vi "(SubVI)Scope_Trigger Counting.vi"(7 "Init":bool, 9 "Sampling Time":dbl format="%#_13g", 10 "Trigger Setting":T1 {"Capture Delay (sec.)" min=0.0 max=5.0; "Pre-Trigger (sec.)" max=10.0}, 11 "Scope Data In":i16[][](array[numeric])) -> (1 "Stop":bool, 2 "Trigger Count":u32, 3 "Scope Data Out":i16[][](array[numeric]))   [LabVIEW 2020]
uses:
  Log/Controls/(Ctrl)Scope_Log_Trigger_Setting.ctl
  Log/Controls/(Ctrl)Scope_Log_Trigger_Type.ctl
  Log/Controls/(Ctrl)Scope_Log_Trigger_Edge.ctl
  Log/Controls/(Ctrl)Scope_Log_Trigger_Edge_Slope.ctl
  Log/Controls/(Ctrl)Scope_Log_Trigger_Window.ctl
  Log/Controls/(Ctrl)Scope_Log_Trigger_Window_When.ctl
  Log/Controls/(Ctrl)Scope_Log_Trigger_Mode.ctl
  a86a7f54-a3bc-428c-973f-614ca024c295.vi
  0bc404e9-e659-4e8a-81b1-d0e0b6e0689e.vi
  <vilib>/Comparison/Equal/Equal Functor/Equal Functor.lvclass
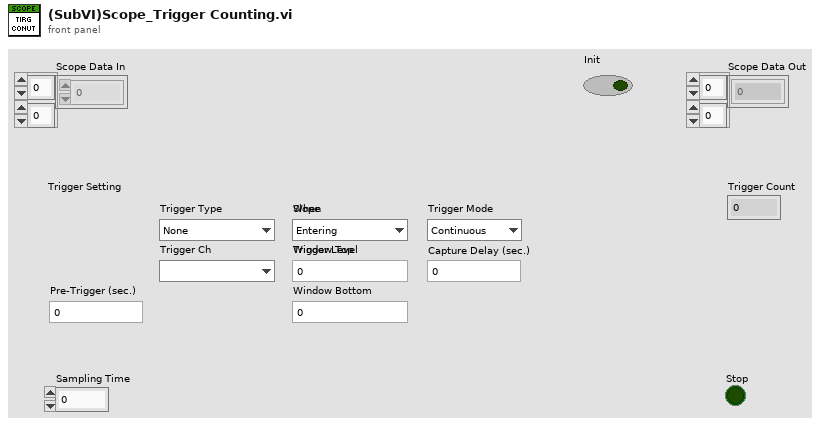
[diagram p1: front panel]
types:
  T1 = typedef "(Ctrl)Scope_Log_Trigger_Setting.ctl" = cluster{"Trigger Type":T2, "Trigger Ch":u16, "Pre-Trigger (sec.)":dbl, "Trigger_Edge":T3, "Trigger_Window":T5, "Trigger Mode":T7, "Capture Delay (sec.)":dbl}
  T2 = typedef "(Ctrl)Scope_Log_Trigger_Type.ctl" = enum16{"None", "Edge", "Window"}
  T3 = typedef "(Ctrl)Scope_Log_Trigger_Edge.ctl" = cluster{"Slope":T4, "Trigger Level":i16}
  T4 = typedef "(Ctrl)Scope_Log_Trigger_Edge_Slope.ctl" = enum16{"Rising", "Falling"}
  T5 = typedef "(Ctrl)Scope_Log_Trigger_Window.ctl" = cluster{"When":T6, "Window Top":i16, "Window Bottom":i16}
  T6 = typedef "(Ctrl)Scope_Log_Trigger_Window_When.ctl" = enum16{"Entering", "Leaving"}
  T7 = typedef "(Ctrl)Scope_Log_Trigger_Mode.ctl" = enum16{"Continuous", "Capture"}
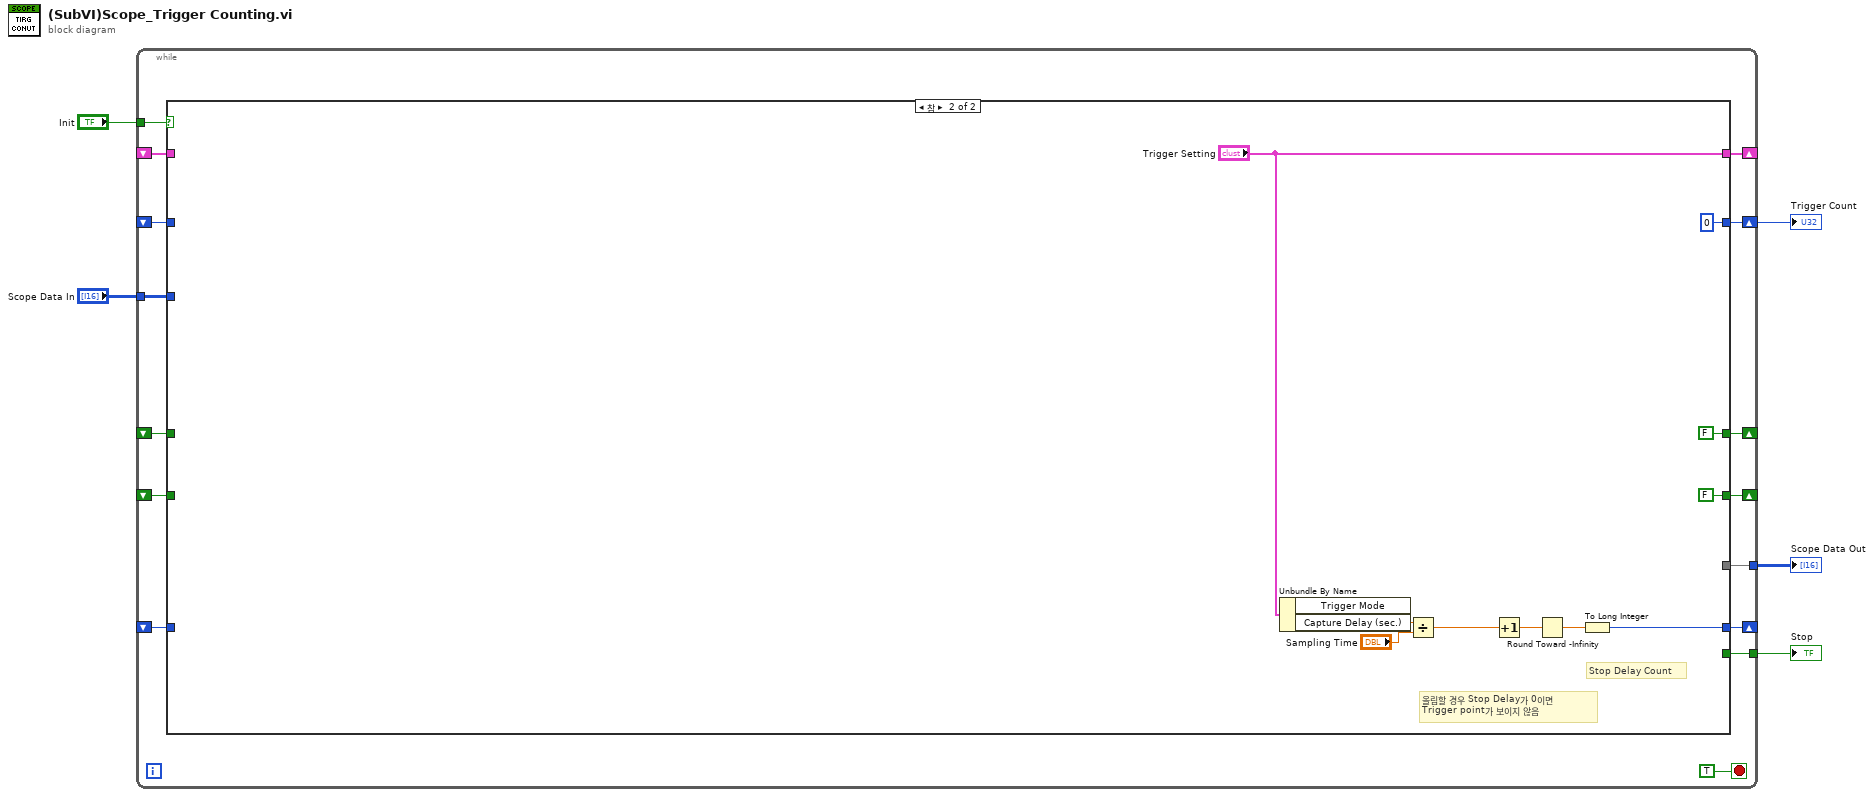
[diagram p0: block diagram]
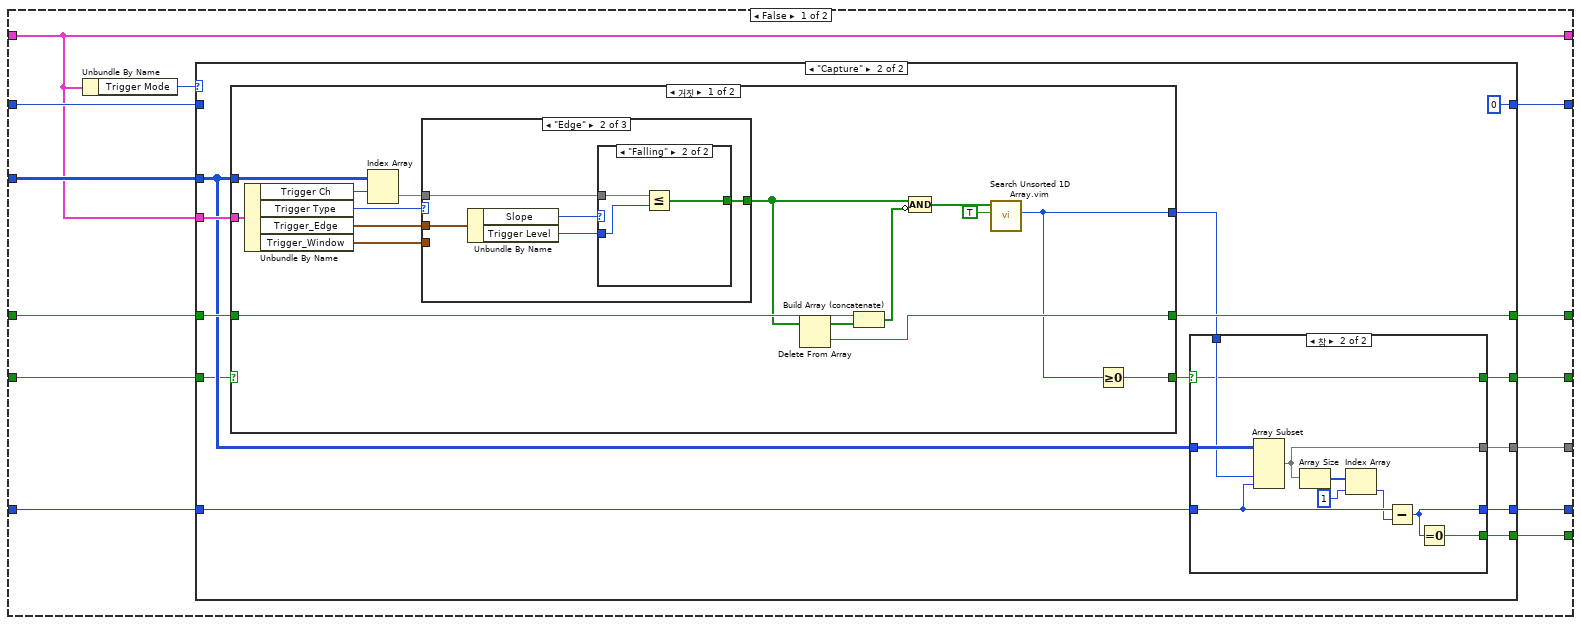
[diagram p2: hidden frame]
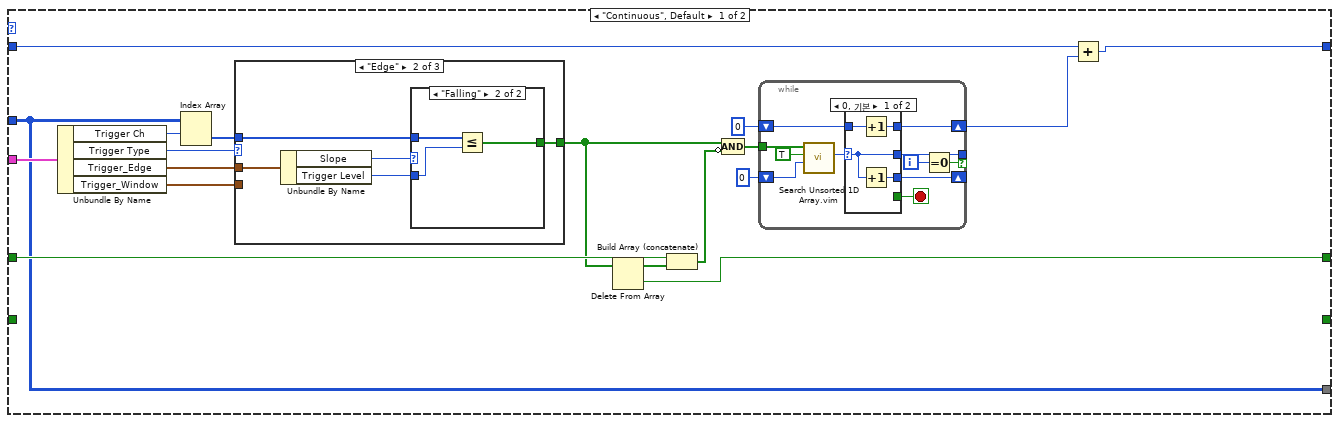
[diagram p3: hidden frame]
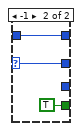
[diagram p4: hidden frame]
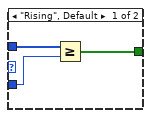
[diagram p6: hidden frame]
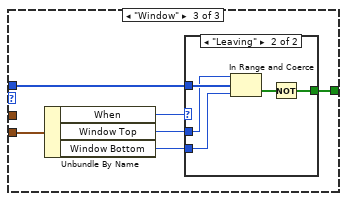
[diagram p7: hidden frame]
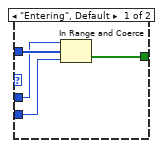
[diagram p8: hidden frame]
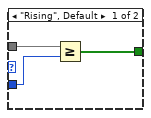
[diagram p10: hidden frame]
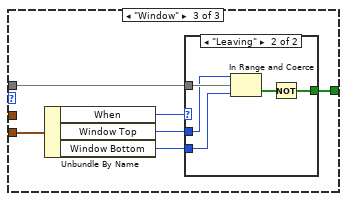
[diagram p11: hidden frame]
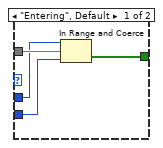
[diagram p12: hidden frame]
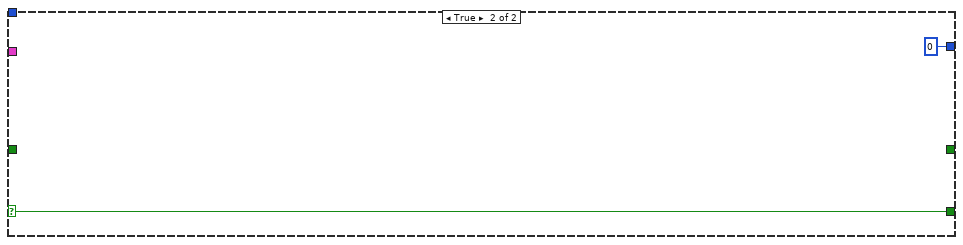
[diagram p13: hidden frame]
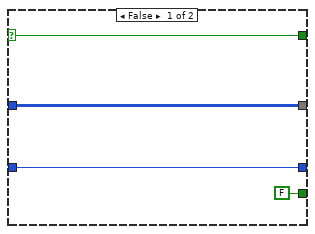
[diagram p14: hidden frame]
diagram:
  n1 = while {
    shift-right: [w20] -> _
    shift-left: _ -> [w19]
    tunnel: "Scope Data In" -> [w15]
    tunnel: "Init" -> [w14]
    shift-right: [w17] -> w1
    shift-left: _ -> [w13]
    shift-right: [w12] -> _
    shift-left: _ -> [w11]
    shift-right: [w10] -> _
    shift-left: _ -> [w16]
    shift-right: [w9] -> _
    shift-left: _ -> [w8]
    tunnel: [w7] -> w3
    tunnel: [w6] -> w2
    stop <- TRUE stop-if-true
    n2 = case shown="참" w14 {
      tunnel: [w33 FALSE ("Window Top")] -> w20
      tunnel: w19 -> [w32 _]
      tunnel: [w30 u32 0] -> w17
      tunnel: w16 -> [w22 _]
      tunnel: w15 -> [w27 _]
      tunnel: w13 -> [w31 _]
      tunnel: [w29 FALSE] -> w12
      tunnel: w11 -> [w28 _]
      tunnel: [w22 "Trigger Setting"] -> w10
      tunnel: [w24 w170] -> w9
      tunnel: w8 -> [w26 _]
      tunnel: [w25 _] -> w7
      tunnel: [w23 _] -> w6
      frame False {
        n3 = Unbundle By Name(w22) -> ("Trigger Mode"=w21:T7)
        n4 = case shown="\"Capture\"" w21 {
          tunnel: [w44 w108] -> w33
          tunnel: w32 -> [w43 w107]
          tunnel: w31 -> [w39 _]
          tunnel: [w38 u32 0] -> w30
          tunnel: [_ w106] -> w29
          tunnel: w28 -> [_ w97]
          tunnel: w22 -> [w36 w104]
          tunnel: w27 -> [w34 w103]
          tunnel: w26 -> [_ w102]
          tunnel: [w34 w101] -> w25
          tunnel: [_ w100] -> w24
          tunnel: [_ w99] -> w23
          frame "Continuous", Default {
            n5 = Unbundle By Name(w36) -> ("Trigger Ch"=w51:u16, "Trigger Type"=w50:T2, "Trigger_Edge"=w48:T3, "Trigger_Window"=w47:T5)
            n6 = Index Array(array=w34, index (row)=w51) -> (element=w49:i16[])  [unwired: 1 in]
            n7 = case shown="\"Edge\"" w50 {
              tunnel: w49 -> [_ w71 w84]
              tunnel: w48 -> [_ w74 _]
              tunnel: w47 -> [_ _ w82]
              tunnel: [_ w70 w83] -> w42
              frame "None" {
              }
              frame "Edge" {
                n8 = Unbundle By Name(w74) -> ("Slope"=w73:T4, "Trigger Level"=w72:i16)
                n9 = case shown="\"Falling\"" w73 {
                  tunnel: w72 -> [w76 w79]
                  tunnel: w71 -> [w77 w80]
                  tunnel: [w75 w78] -> w70
                  frame "Rising", Default {
                    n10 = Greater Or Equal?(x=w77, y=w76) -> (x >= y?=w75:bool[])
                  }
                  frame "Falling" {
                    n11 = Less Or Equal?(x=w80, y=w79) -> (x <= y?=w78:bool[])
                  }
                }
              }
              frame "Window" {
                n12 = Unbundle By Name(w82) -> ("When"=w86:T6, "Window Top"=w85:i16, "Window Bottom"=w81:i16)
                n13 = case shown="\"Leaving\"" w86 {
                  tunnel: w85 -> [w88 w93]
                  tunnel: w84 -> [w89 w94]
                  tunnel: [w90 w91] -> w83
                  tunnel: w81 -> [w87 w92]
                  frame "Entering", Default {
                    n14 = In Range and Coerce(upper limit=w88, x=w89, lower limit=w87) -> (In Range?=w90:bool[])  [unwired: 1 out]
                  }
                  frame "Leaving" {
                    n15 = In Range and Coerce(upper limit=w93, x=w94, lower limit=w92) -> (In Range?=w95:bool[])  [unwired: 1 out]
                    n16 = Not(x=w95) -> (.not. x?=w91:bool[])
                  }
                }
              }
            }
            n17 = Delete From Array(array=w42) -> (deleted portion=w44:bool, array with subset deleted=w45:bool[])  [unwired: 2 in]
            n18 = Build Array (concatenate)(w43, w45) -> (w46:bool[])
            n19 = Compound Arithmetic op=AND(w42, invert w46) -> (w41:bool[])
            n20 = while {
              tunnel: w41 -> [w61]
              shift-right: [w59] -> _
              shift-left: 0 -> [w58]
              shift-right: [w55] -> w37
              shift-left: u32 0 -> [w56]
              tunnel: [w54] -> _ if=w53
              i -> [w52]
              stop <- w57 stop-if-true
              n21 = call "Search Unsorted 1D Array.vim"("start index (0)"=w58, "element"=TRUE, "unsorted 1D array"=w61) -> ("index of element"=w60:i32)  [unwired: 8 in]
              n22 = case shown="0, 기본" w60 {
                selector: w60 -> [w63 w67]
                tunnel: [w66 _] -> w59
                tunnel: [_ TRUE] -> w57
                tunnel: w56 -> [w65 w68]
                tunnel: [w64 w68] -> w55
                tunnel: [w63 w67] -> w54
                frame 0, Default {
                  n23 = Increment(x=w65) -> (x+1=w64:u32)
                  n24 = Increment(x=w63) -> (x+1=w66:i32)
                }
                frame -1 {
                }
              }
              n25 = Equal To 0?(x=w52) -> (x = 0?=w53:bool)
            }
            n26 = Add(x=w39, y=w37) -> (x+y=w38:u32)
          }
          frame "Capture" {
            n27 = case shown="거짓" w97 {
              selector: w97 -> [_ w151]
              tunnel: [w117 _] -> w108
              tunnel: w107 -> [w116 _]
              tunnel: [w110 0 ("index of element")] -> w105
              tunnel: w104 -> [w113 _]
              tunnel: w103 -> [w112 _]
              tunnel: [w109 w151] -> w96
              frame False {
                n28 = Unbundle By Name(w113) -> ("Trigger Ch"=w124:u16, "Trigger Type"=w123:T2, "Trigger_Edge"=w121:T3, "Trigger_Window"=w120:T5)
                n29 = Index Array(array=w112, index (row)=w124) -> (element=w122:i16[])  [unwired: 1 in]
                n30 = case shown="\"Edge\"" w123 {
                  tunnel: w122 -> [_ w126 w139]
                  tunnel: w121 -> [_ w129 _]
                  tunnel: w120 -> [_ _ w137]
                  tunnel: [_ w125 w138] -> w115
                  frame "None" {
                  }
                  frame "Edge" {
                    n31 = Unbundle By Name(w129) -> ("Slope"=w128:T4, "Trigger Level"=w127:i16)
                    n32 = case shown="\"Falling\"" w128 {
                      tunnel: w127 -> [w131 w134]
                      tunnel: w126 -> [w132 w135]
                      tunnel: [w130 w133] -> w125
                      frame "Rising", Default {
                        n33 = Greater Or Equal?(x=w132, y=w131) -> (x >= y?=w130:bool[])
                      }
                      frame "Falling" {
                        n34 = Less Or Equal?(x=w135, y=w134) -> (x <= y?=w133:bool[])
                      }
                    }
                  }
                  frame "Window" {
                    n35 = Unbundle By Name(w137) -> ("When"=w141:T6, "Window Top"=w140:i16, "Window Bottom"=w136:i16)
                    n36 = case shown="\"Leaving\"" w141 {
                      tunnel: w140 -> [w143 w148]
                      tunnel: w139 -> [w144 w149]
                      tunnel: [w145 w146] -> w138
                      tunnel: w136 -> [w142 w147]
                      frame "Entering", Default {
                        n37 = In Range and Coerce(upper limit=w143, x=w144, lower limit=w142) -> (In Range?=w145:bool[])  [unwired: 1 out]
                      }
                      frame "Leaving" {
                        n38 = In Range and Coerce(upper limit=w148, x=w149, lower limit=w147) -> (In Range?=w150:bool[])  [unwired: 1 out]
                        n39 = Not(x=w150) -> (.not. x?=w146:bool[])
                      }
                    }
                  }
                }
                n40 = Delete From Array(array=w115) -> (deleted portion=w117:bool, array with subset deleted=w118:bool[])  [unwired: 2 in]
                n41 = Build Array (concatenate)(w116, w118) -> (w119:bool[])
                n42 = Compound Arithmetic op=AND(w115, invert w119) -> (w114:bool[])
                n43 = call "Search Unsorted 1D Array.vim"("element"=TRUE, "unsorted 1D array"=w114) -> ("index of element"=w110:i32)  [unwired: 9 in]
                n44 = Greater Or Equal To 0?(x=w110) -> (x >= 0?=w109:bool)
              }
              frame True {
              }
            }
            n45 = case shown="참" w96 {
              selector: w96 -> [w154 w160]
              tunnel: [w154 w160] -> w106
              tunnel: w105 -> [_ w164]
              tunnel: w103 -> [w155 w166]
              tunnel: w102 -> [w156 w165]
              tunnel: [w156 w158] -> w100
              tunnel: [w155 w163] -> w101
              tunnel: [FALSE w157] -> w99
              frame False {
              }
              frame True {
                n46 = Array Subset(array=w166, index (col)=w164, length (col)=w165) -> (w163:i16[][])  [unwired: 2 in]
                n47 = Array Size(array=w163) -> (size(s)=w162:i32[])
                n48 = Index Array(array=w162, index=1 ("인덱스")) -> (element=w161:i32)
                n49 = Subtract(x=w165, y=w161) -> (x-y=w158:i32)
                n50 = Equal To 0?(x=w158) -> (x = 0?=w157:bool)
              }
            }
          }
        }
      }
      frame True {
        # "올림할 경우 Stop Delay가 0이면\nTrigger point가 보이지 않음"
        # "Stop Delay Count"
        n51 = Unbundle By Name("Trigger Setting") -> ("Capture Delay (sec.)"=w172:dbl)  [unwired: 1 out]
        n52 = Divide(x=w172, y="Sampling Time") -> (x/y=w169:dbl)
        n53 = Increment(x=w169) -> (x+1=w168:dbl)
        n54 = Round Toward -Infinity(1:w168) -> (0:w167:dbl)
        n55 = To Long Integer(number=w167) -> (32bit integer=w170:i32)
      }
    }
  }
  "Trigger Count" <- w1
  "Scope Data Out" <- w3
  "Stop" <- w2
